vi "PUT Minimum Output Voltage.vi"(0 "Minimum Output Voltage":dbl) -> ()   [LabVIEW 2013]
uses:
  Action.ctl
  Physical Constants FGV Selector.ctl
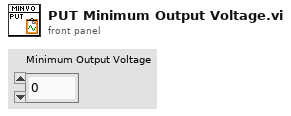
[diagram p1: front panel]
types:
  T1 = typedef "Physical Constants FGV Selector.ctl" = enum16{"Maximum Output Voltage", "Minimum Output Voltage", "Maximum Input Voltage", "Minimum Input Voltage"}
  T2 = typedef "Action.ctl" = enum16{"GET", "PUT", "DELETE"}
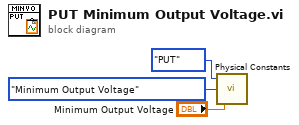
[diagram p0: block diagram]
diagram:
  n1 = call "Physical Constants.vi"("Input"="Minimum Output Voltage", "Physical Constants FGV Selector"=Physical_Constants_FGV_Selector."Minimum Output Voltage", "Action"=Action."PUT") -> ()  [unwired: 1 out]
